vi "Digital to Analog Latency Tester.vi"() -> ()   [LabVIEW 2013]
doc: "This is the FPGA VI for the 10-Tap 8-Bit Camera with DRAM example. This example demonstrates how to acquire images from a 10-tap, 8-bit, extended configuration, Camera Link camera and transfer the images to the host. This example supports area scan and line scan cameras for both continuous and finite acquisitions.\n\nThis example also demonstrates the use of DRAM as a frame buffer for very high speed acquisitions. Data packing and flow-control are also employed to maximize use of the available DRAM and FIFOs in terms of both memory space and performance.\n\nAdditionally, the example demonstrates the serial server, which allows third-party camera configuration utilities to communicate with the camera using the Camera Link serial interface while this VI is running."
uses:
  <vilib>/Platform/TimedLoop/XDataNode/timing_clust.ctl
  <vilib>/Platform/TimedLoop/XDataNode/nitl_modes.ctl
  <vilib>/Platform/TimedLoop/XDataNode/wakeup.ctl
  <vilib>/rvi/Emulation/niFpgaSctlEmulationGetInTimedLoop.vi
  <vilib>/rvi/Emulation/niFpgaEmulationReportErrorSimple.vi
  <vilib>/rvi/Emulation/niFpgaGetClockAttributes.vi
  <vilib>/rvi/Emulation/niFpgaCriticalErrorInLSC.vi
  <vilib>/rvi/eio/common/nirviEmuTemplateMethod_errors.vi
  <vilib>/Platform/TimedLoop/XDataNode/XDataNode.xnode
  <vilib>/eio/EIONode/EIONode.xnode
  <vilib>/Platform/TimedLoop/XDataNode/XDNodeRunTimeDep.lvlib
panel:
  in  "On":bool
  out "Ticks Elapsed":u32
  out "Time PWM Set":u32 caption="Tick Count(Ticks)"
  in  "frequency (periods/tick)":fxp<+,32,0>=2.500019036233425e-05 caption="frequency"
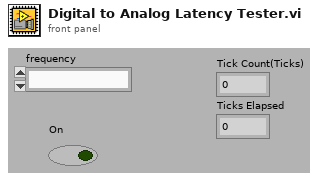
[diagram p1: front panel]
types:
  T1 = typedef "XDNodeRunTimeDep.lvlib/timing_clust.ctl" = cluster{"Expected End [f-1]":u64, "Actual End [f-1]":u64, "Finished Late? [f-1]":bool, "Expected End [i-1]":u64, "Actual End [i-1]":u64, "Finished Late? [i-1]":bool, "Expected Start [i]":u64, "Actual Start [i]":u64, "Expected Start [f]":u64, "Actual Start [f]":u64, "Source Name":string, "Structure Name":string, "Period":i64, "Deadline":i64, "Offset":i64, "Start":i64, "Priority":i32, "Timeout":i32, "Mode":T2, "Wakeup Reason":T3, "Error":errorcluster, "Source Type":string, "Secondary Source Type":string, "Global End Time":u64, "Global Start Time":u64, "Frame Duration":u64, "Iteration Duration":u64, "Assigned CPU":i32, "I/O Scan Engine Mode":u32}
  T2 = typedef "XDNodeRunTimeDep.lvlib/nitl_modes.ctl" = enum32{"No Change", "Process missed periods, maintain original phase", "Discard missed periods, maintain original phase", "Process missed periods, ignore original phase", "Discard missed periods, ignore original phase"}
  T3 = typedef "XDNodeRunTimeDep.lvlib/wakeup.ctl" = enum32{"Normal", "Aborted", "Asynchronous wakeup", "Timing source error", "Timed loop error", "Timeout"}
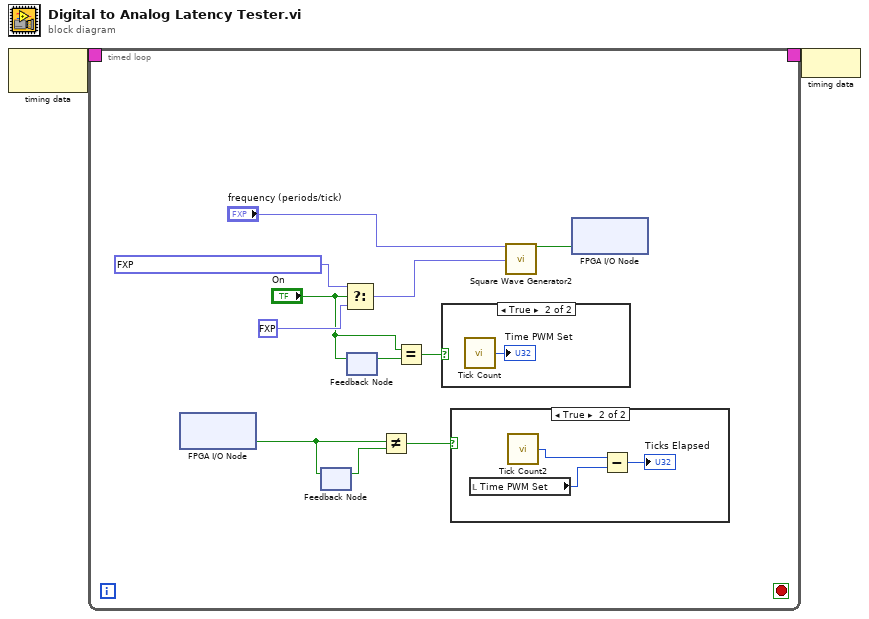
[diagram p0: block diagram]
diagram:
  n1 = node-c288() -> (w2:T1)  [unwired: 1 in]
  n2 = timed-loop {
    timing: w2 -> [_]
    timing-out: [_] -> w1
    stop <- _ stop-if-true
    n3 = xnode "FPGA I/O Node"() -> ("TTL 1"=w11:bool)  [unwired: 1 in, 1 out]
    n4 = feedback #1() -> (w12:bool)  [unwired: 1 in]
    n5 = feedback-in #1(w11) -> ()
    n6 = Select(t=fxp<+,32,0> 0.9999999997671694 ("duty cycle (periods)"), s="On", f=fxp<+,32,0> 0.0 ("duty cycle (periods)")) -> (s? t:f=w6:fxp<+,32,0>)
    n7 = feedback #2() -> (w5:bool)  [unwired: 1 in]
    n8 = feedback-in #2("On") -> ()
    n9 = Not Equal?(x=w11, y=w12) -> (x != y?=w13:bool)
    n10 = Equal?(x="On", y=w5) -> (x = y?=w3:bool)
    n11 = case shown="True" w3 {
      frame False {
      }
      frame True {
        n12 = call "Tick Count"() -> ("Tick Count(Ticks)"=→"Time PWM Set":u32)
      }
    }
    n13 = case shown="True" w13 {
      frame False {
      }
      frame True {
        n14 = local read "Time PWM Set"() -> (w16:u32)
        n15 = call "Tick Count2"() -> ("Tick Count(Ticks)"=w17:u32)
        n16 = Subtract(x=w17, y=w16) -> (x-y=→"Ticks Elapsed":u32)
      }
    }
    n17 = call "Square Wave Generator2"("frequency (periods/tick)"="frequency (periods/tick)", "duty cycle (periods)"=w6) -> ("square wave out"=w9:bool)  [unwired: 13 in]
    n18 = xnode "FPGA I/O Node"("TTL 0"=w9) -> ()  [unwired: 1 in, 1 out]
  }
  n19 = node-c288(w1) -> ()
